vi "TermLoopBack.vi"(3 "error in (no error)":errorcluster {"code" format="%.0x"}, 4 "topology name":T1="2566/16-SPDT", 5 "PXI resource name":refnum<k15>="PXI1Slot6", 6 "VISA resource name":refnum<visa-resource-name>="COM1") -> (0 "error out":errorcluster, 1 "Receive_buffer":u8[](array[numeric]) format="%x", 2 "VISA resource name Out":refnum<visa-resource-name>)   [LabVIEW 2014]
uses:
  <instrlib>/niSwitch/niswitch.llb/niSwitch Topologies.ctl
panel:
  out "Read Count 2":u32
  out "Receive_buffer 2":u8[](array[numeric]) format="%x"
  out "Read Count":u32
  out "Write Count":u32
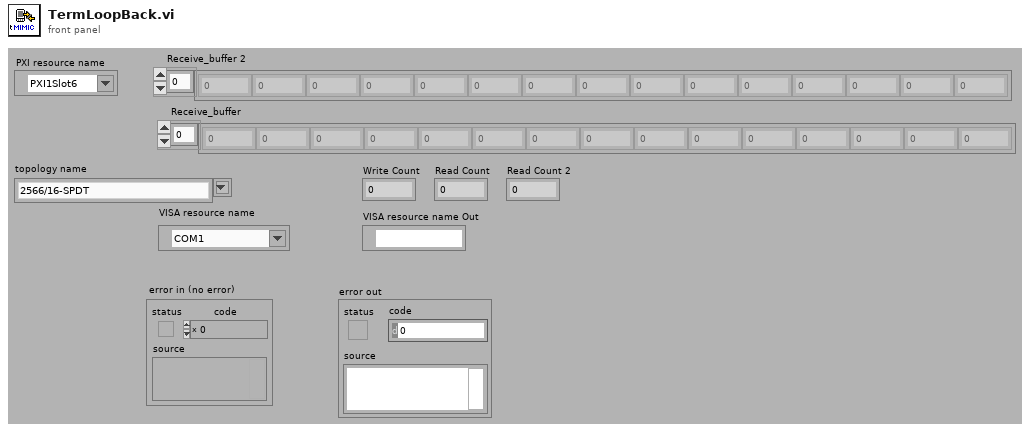
[diagram p1: front panel]
types:
  T1 = typedef "niSwitch Topologies.ctl" = string
  T2 = enum16{"Init Control Relays", "Secondary RS232", "Term Loopback", "CTS Isolate", "Synapse Loopback", "CST RTS Loopback", "Command Flash", "Auxillary RS232", "Battery Charge", "Remote Power", "Cordless Boot", "Auxillary Port", "DeInit Control Relays"}
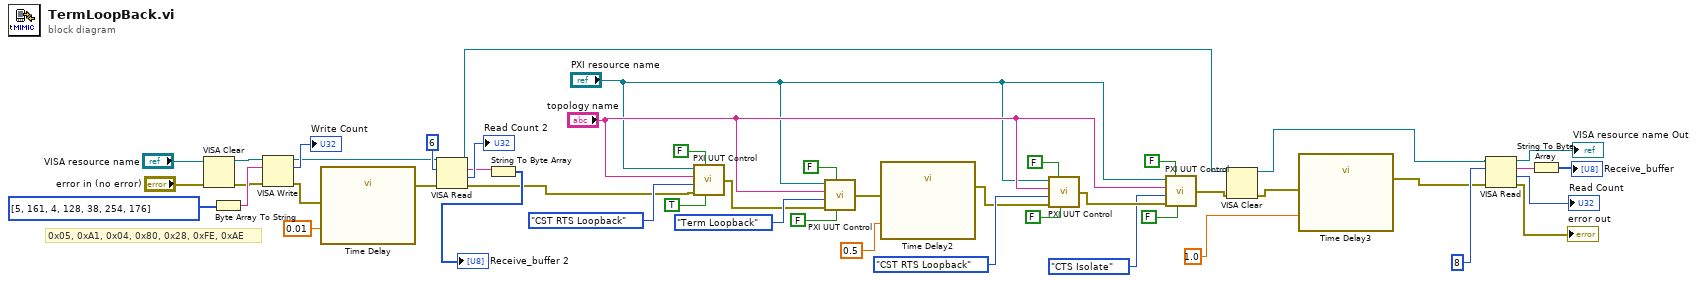
[diagram p0: block diagram]
diagram:
  # "0x05, 0xA1, 0x04, 0x80, 0x28, 0xFE, 0xAE"
  n1 = VISA Clear(VISA resource name="VISA resource name", error in (no error)="error in (no error)") -> (VISA resource name out=w29:refnum<visa-resource-name>, error out=w30:errorcluster)
  n2 = Byte Array To String(unsigned byte array=u8[] [5, 161, 4, 128, 38, 254, 176] ("Command array")) -> (string=w45:string)
  n3 = VISA Write(VISA resource name=w29, write buffer=w45, error in (no error)=w30) -> (VISA resource name out=w24:refnum<visa-resource-name>, return count=→"Write Count":u32, error out=w23:errorcluster)
  n4 = call "Time Delay"("error in (no error)"=w23, "Delay Time (s)"=0.01) -> ("error out"=w22:errorcluster)  [unwired: 9 in]
  n5 = VISA Read(VISA resource name=w24, byte count=u32 6, error in (no error)=w22) -> (VISA resource name out=w5:refnum<visa-resource-name>, read buffer=w26:string, return count=→"Read Count 2":u32, error out=w1:errorcluster)
  n6 = String To Byte Array(string=w26) -> (unsigned byte array=→"Receive_buffer 2":u8[])
  n7 = call "PXI UUT Control.vi"("Enable Relays"=TRUE, "Reset IO"=FALSE, "error in (no error)"=w1, "Enum"=T2."CST RTS Loopback", "topology name"="topology name", "resource name"="PXI resource name") -> ("error out"=w13:errorcluster)
  n8 = call "PXI UUT Control.vi"("Enable Relays"=FALSE, "Reset IO"=FALSE, "error in (no error)"=w13, "Enum"=T2."Term Loopback", "topology name"="topology name", "resource name"="PXI resource name") -> ("error out"=w20:errorcluster)
  n9 = call "Time Delay2"("error in (no error)"=w20, "Delay Time (s)"=0.5) -> ("error out"=w19:errorcluster)  [unwired: 9 in]
  n10 = call "PXI UUT Control.vi"("Enable Relays"=FALSE, "Reset IO"=FALSE, "error in (no error)"=w19, "Enum"=T2."CST RTS Loopback", "topology name"="topology name", "resource name"="PXI resource name") -> ("error out"=w8:errorcluster)
  n11 = call "PXI UUT Control.vi"("Enable Relays"=FALSE, "Reset IO"=FALSE, "error in (no error)"=w8, "Enum"=T2."CTS Isolate", "topology name"="topology name", "resource name"="PXI resource name") -> ("error out"=w6:errorcluster)
  n12 = VISA Clear(VISA resource name=w5, error in (no error)=w6) -> (VISA resource name out=w4:refnum<visa-resource-name>, error out=w2:errorcluster)
  n13 = call "Time Delay3"("error in (no error)"=w2, "Delay Time (s)"=1.0) -> ("error out"=w3:errorcluster)  [unwired: 9 in]
  n14 = VISA Read(VISA resource name=w4, byte count=u32 8, error in (no error)=w3) -> (VISA resource name out=→"VISA resource name Out":refnum<visa-resource-name>, read buffer=w40:string, return count=→"Read Count":u32, error out=→"error out":errorcluster)
  n15 = String To Byte Array(string=w40) -> (unsigned byte array=→"Receive_buffer":u8[])
